vi "DIFF_DRIVE_KINEMATIC_FGV.vi"(8 "in DIFF_DRIVE_KINEMATICS":T1 {"TrackWidth_Meters" format="%20.4f"}, 11 "Write":bool) -> (0 "out DIFF_DRIVE_KINEMATICS":T1 {"TrackWidth_Meters" format="%20.4f"})   [LabVIEW 2023]
uses:
  <vilib>/Rock Robotics/WPI/ThirdParty/JAS_Junk/TrajLib/TypeDef/DIFF_DRIVE_KINEMATICS.ctl
  <vilib>/Rock Robotics/WPI/ThirdParty/JAS_Junk/TrajLib/Trajectory_Library.lvlib
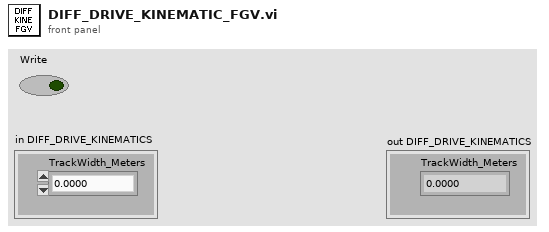
[diagram p1: front panel]
types:
  T1 = typedef "Trajectory_Library.lvlib/DIFF_DRIVE_KINEMATICS.ctl" = cluster{"TrackWidth_Meters":dbl}
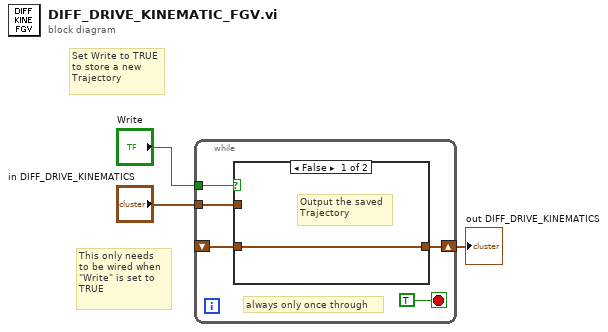
[diagram p0: block diagram]
diagram:
  # "This only needs\nto be wired when\n\"Write\" is set to\nTRUE"
  # "Set Write to TRUE\nto store a new\nTrajectory"
  n1 = while {
    tunnel: "Write" -> [w7]
    tunnel: "in DIFF_DRIVE_KINEMATICS" -> [w5]
    shift-right: [w6] -> w1
    shift-left: _ -> [w4]
    stop <- TRUE stop-if-true
    # "always only once through"
    n2 = case shown="False" w7 {
      tunnel: [w9 w10] -> w6
      tunnel: w5 -> [_ w10]
      tunnel: w4 -> [w9 _]
      frame False {
        # "Output the saved\nTrajectory"
      }
      frame True {
        # "Save the trajectory\nin the shift \nregister."
      }
    }
  }
  "out DIFF_DRIVE_KINEMATICS" <- w1
